vi "Attempt Connect.vi"(8 "error in (no error)":errorcluster, 10 "Seconds to attempt":i32, 11 "Refnum in":refnum<k21>) -> (0 "error out":errorcluster)   [LabVIEW 2012, in "PXImc Engine.lvlib"]
uses:
  PXImc Engine.lvlib
  <vilib>/pximc/Connect (DBL).vi
  <vilib>/pximc/nipximc.lvlib
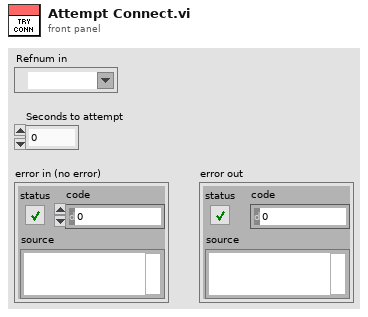
[diagram p1: front panel]
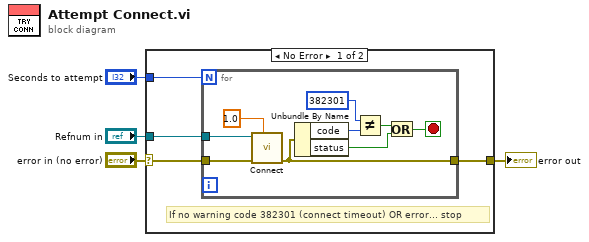
[diagram p0: block diagram]
diagram:
  n1 = case shown="No Error" "error in (no error)" {
    selector: "error in (no error)" -> [w5 w18]
    tunnel: [w8 w18] -> w4
    tunnel: "Seconds to attempt" -> [w7 _]
    tunnel: "Refnum in" -> [w6 _]
    frame No Error {
      # "If no warning code 382301 (connect timeout) OR error... stop"
      n2 = for {
        N: w7 -> [_]
        tunnel: w5 -> [w17]
        tunnel: w6 -> [w16]
        tunnel: [w9] -> w8
        stop <- w10 stop-if-true
        n3 = call-poly <vilib>:"Connect.vi"("timeout in seconds (-1)"=1.0, "error in (no error)"=w17, "session in"=w16) -> ("error out"=w9:errorcluster)  [unwired: 7 in, 1 out]
        n4 = Unbundle By Name(w9) -> ("code"=w13:i32, "status"=w14:bool)
        n5 = Not Equal?(x=382301, y=w13) -> (x != y?=w11:bool)
        n6 = Or(x=w11, y=w14) -> (x .or. y?=w10:bool)
      }
    }
    frame Error {
    }
  }
  "error out" <- w4
